vi "Configure Reference.vi"(0 "VISA resource name":refnum<visa-resource-name>, 1 "Detection Harmonic Number (1)":dbl=1.0, 2 "Internal Reference Frequency (100000Hz)":dbl=100000.0, 5 "Reference Source (0: Internal)":i32(ring) items=["Internal", "External", "Dual", "Chop"], 7 "Manual Phase (0 Degree)":dbl, 9 "Auto Phase(0:Disabled)":bool, 11 "error in (no error)":errorcluster, 12 "External Reference Trigger (0: Sine Zero Crossing)":i32(ring) items=["Sine Zero Crossing", "Positive TTL", "Negative TTL"], 13 "External Reference Trigger Input (0: 50OHMS)":i32(ring) items=["50OHMS", "1megaOHMS"]) -> (4 "VISA resource name out":refnum<visa-resource-name>)   [LabVIEW 2020, in "Stanford Research SR865.lvlib"]
doc: "Configures the reference source and the internal oscillator."
uses:
  Stanford Research SR865.lvlib
panel:
  # "Internal Reference Trigger"
  # "External Reference Trigger"
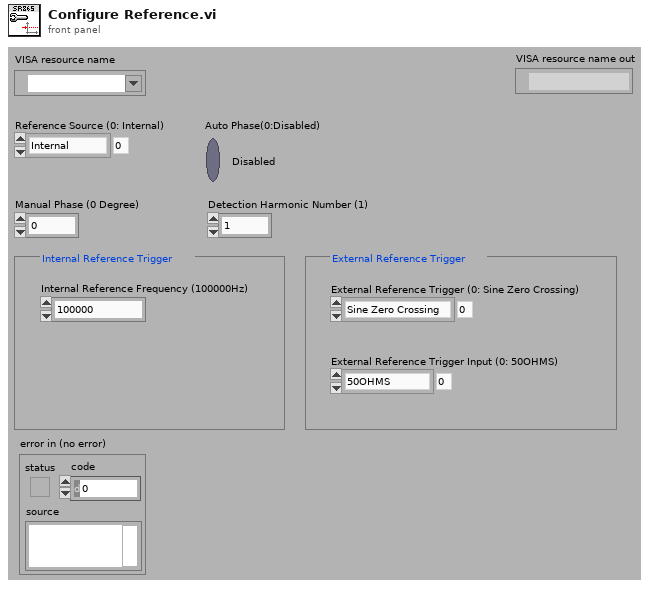
[diagram p1: front panel]
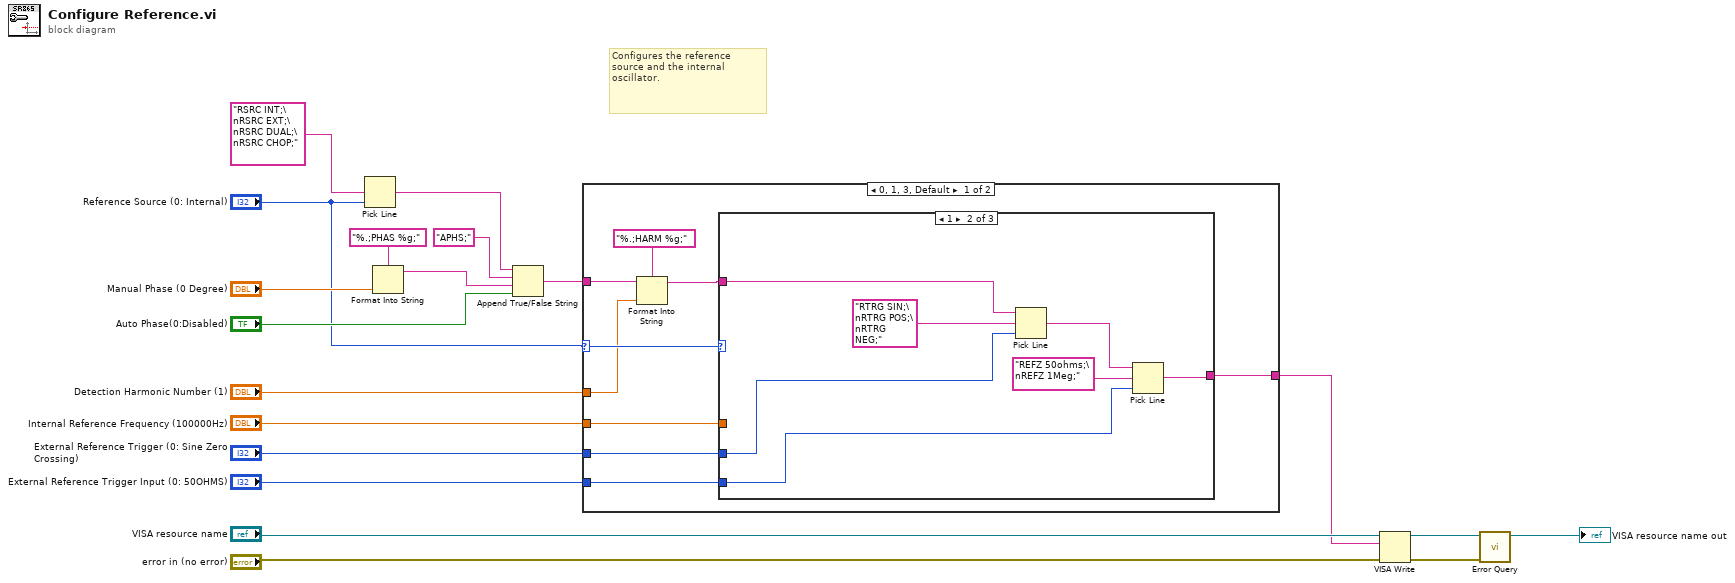
[diagram p0: block diagram]
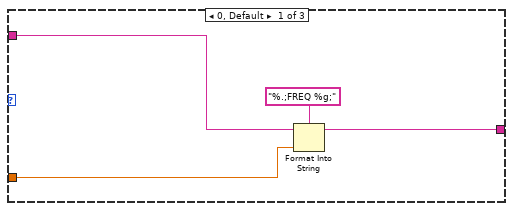
[diagram p2: hidden frame]
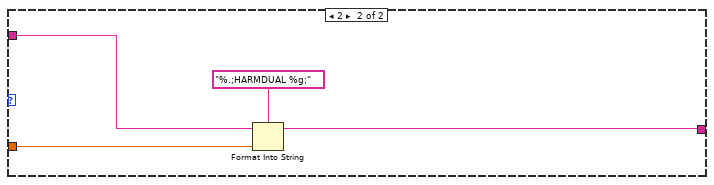
[diagram p4: hidden frame]
diagram:
  # "Configures the reference source and the internal oscillator."
  n1 = Pick Line(multi-line string="RSRC INT;\nRSRC EXT;\nRSRC DUAL;\nRSRC CHOP;", line index="Reference Source (0: Internal)") -> (output string=w9:string)  [unwired: 1 in]
  n2 = Format Into String(format string="%.;PHAS %g;", "Manual Phase (0 Degree)") -> (resulting string=w11:string)  [unwired: 2 in, 1 out]
  n3 = Append True/False String(1:"Auto Phase(0:Disabled)", 2:w11, 3:"APHS;", 4:w9) -> (0:w8:string)
  n4 = case shown="0, 1, 3, Default" "Reference Source (0: Internal)" {
    selector: "Reference Source (0: Internal)" -> [w28 _]
    tunnel: w8 -> [w25 w43]
    tunnel: "Detection Harmonic Number (1)" -> [w23 w42]
    tunnel: [w27 w41] -> w4
    tunnel: "Internal Reference Frequency (100000Hz)" -> [w22 _]
    tunnel: "External Reference Trigger (0: Sine Zero Crossing)" -> [w21 _]
    tunnel: "External Reference Trigger Input (0: 50OHMS)" -> [w20 _]
    frame 0, 1, 3, Default {
      n5 = Format Into String(format string="%.;HARM %g;", initial string=w25, w23) -> (resulting string=w24:string)  [unwired: 1 in, 1 out]
      n6 = case shown="1" w28 {
        tunnel: w24 -> [w31 w35 w40]
        tunnel: [w30 w36 w40] -> w27
        tunnel: w22 -> [w29 _ _]
        tunnel: w21 -> [_ w34 _]
        tunnel: w20 -> [_ w33 _]
        frame 0, Default {
          n7 = Format Into String(format string="%.;FREQ %g;", initial string=w31, w29) -> (resulting string=w30:string)  [unwired: 1 in, 1 out]
        }
        frame 1 {
          n8 = Pick Line(string ("")=w35, multi-line string="RTRG SIN;\nRTRG POS;\nRTRG NEG;", line index=w34) -> (output string=w39:string)
          n9 = Pick Line(string ("")=w39, multi-line string="REFZ 50ohms;\nREFZ 1Meg;", line index=w33) -> (output string=w36:string)
        }
        frame 3 {
        }
      }
    }
    frame 2 {
      n10 = Format Into String(format string="%.;HARMDUAL %g;", initial string=w43, w42) -> (resulting string=w41:string)  [unwired: 1 in, 1 out]
    }
  }
  n11 = VISA Write(VISA resource name="VISA resource name", write buffer=w4, error in (no error)="error in (no error)") -> (VISA resource name out=w15:refnum<visa-resource-name>, error out=w14:errorcluster)  [unwired: 1 out]
  n12 = call "Error Query.vi"("error in (no error)"=w14, "VISA resource name"=w15) -> ("VISA resource name out"=→"VISA resource name out":refnum<visa-resource-name>)  [unwired: 7 in, 2 out]
